vi "NanoStep Goto.vi"(0 "VISA Rsrc":refnum<visa-resource-name>="GPIB1::15::INSTR", 1 "AxeInv":bool, 5 "Position":dbl=0.5, 7 "Input Units":i8(ring) items=["mm", "ps"], 9 "Axis":u16(ring)=1 items=["Axis 0", "Axis 1"], 11 "error in":errorcluster, 12 "CtrlRef":T1 caption="Control Reference") -> (6 "Pos Out":dbl=0.5, 15 "error out":errorcluster)   [LabVIEW 2010]
uses:
  <userlib>/GenProg/WritebyRefBool.vi
  <userlib>/GenProg/ReadbyRefBool.vi
  <userlib>/GenProg/WritebyRefNum.vi
panel:
  in  "Annuler":bool
  out "Init Done":bool
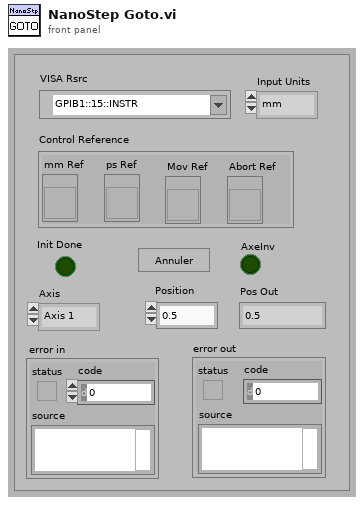
[diagram p1: front panel]
types:
  T1 = cluster{"mm Ref":refnum<vi>, "ps Ref":refnum<vi>, "Mov Ref":refnum<vi>, "Abort Ref":refnum<vi>}
  T2 = enum16{"send command", "Init axis", "read position", "read limit", "end"}
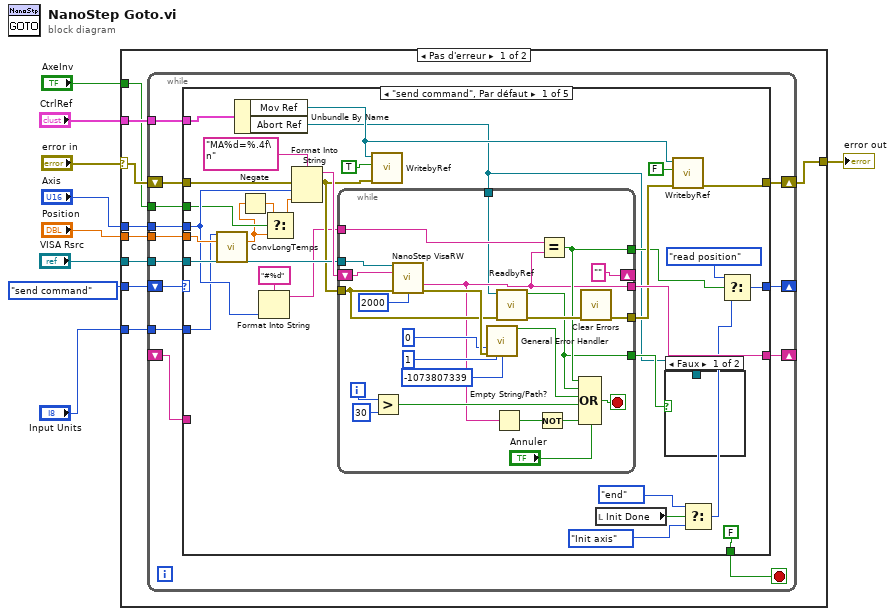
[diagram p0: block diagram]
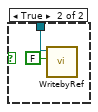
[diagram p2: hidden frame]
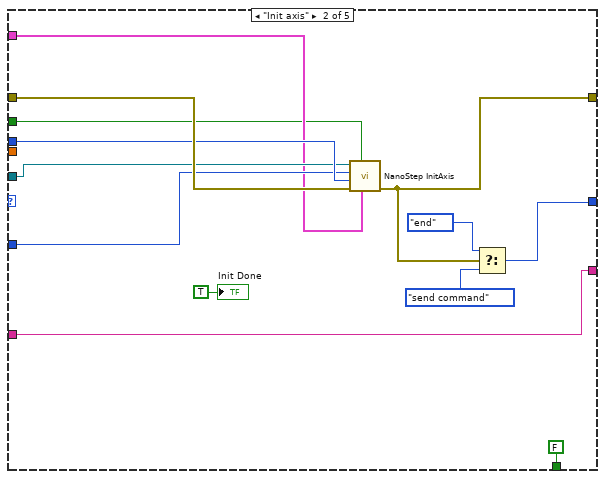
[diagram p3: hidden frame]
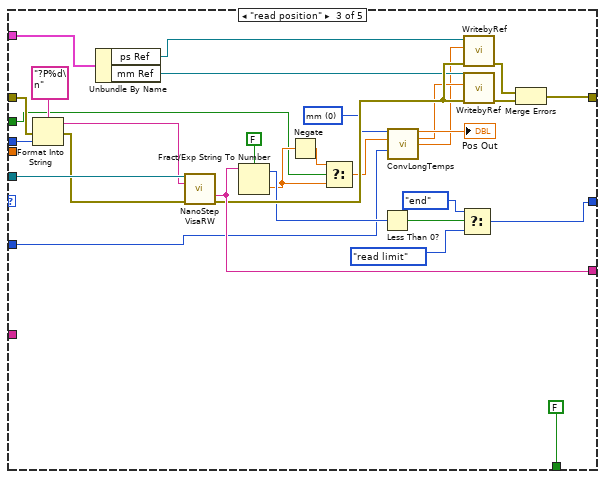
[diagram p4: hidden frame]
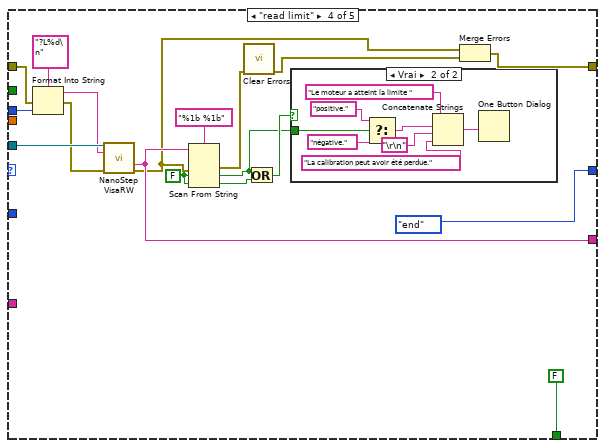
[diagram p5: hidden frame]
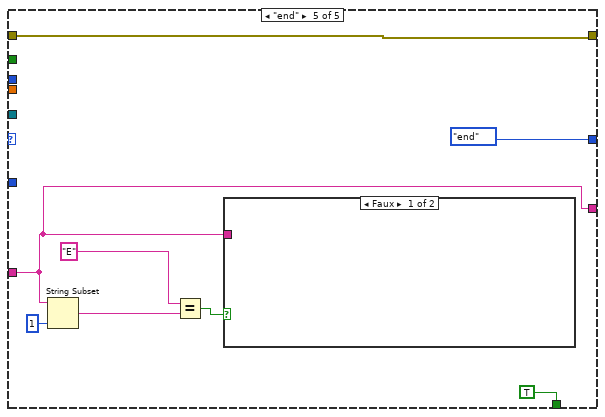
[diagram p7: hidden frame]
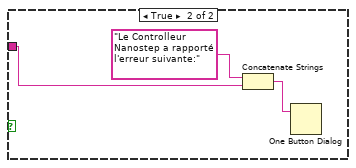
[diagram p8: hidden frame]
diagram:
  n1 = case shown="Pas d'erreur" "error in" {
    selector: "error in" -> [w15 w169]
    tunnel: "Axis" -> [w17 _]
    tunnel: "Position" -> [w18 _]
    tunnel: [w14 w169] -> w6
    tunnel: T2."send command" ("Énum") -> [w16 _]
    tunnel: "VISA Rsrc" -> [w13 _]
    tunnel: "Input Units" -> [w12 _]
    tunnel: "CtrlRef" -> [w11 _]
    tunnel: "AxeInv" -> [w10 _]
    frame No Error {
      n2 = while {
        tunnel: w18 -> [w31]
        tunnel: w17 -> [w30]
        shift-right: [w26] -> w14
        shift-left: w15 -> [w28]
        tunnel: w13 -> [w27]
        shift-right: [w24] -> _
        shift-left: w16 -> [w29]
        shift-right: [w23] -> _
        shift-left: _ -> [w22]
        tunnel: w12 -> [w21]
        tunnel: w11 -> [w20]
        tunnel: w10 -> [w19]
        stop <- w25 stop-if-true
        n3 = case shown="\"send command\", Par défaut" w29 {
          tunnel: w31 -> [w53 _ _ _ _]
          tunnel: w30 -> [w45 w100 w129 w147 _]
          tunnel: w28 -> [w61 w101 w128 w146 w161]
          tunnel: w27 -> [w57 w98 w131 w149 _]
          tunnel: [w51 w97 w120 w137 w161] -> w26
          tunnel: [FALSE FALSE FALSE FALSE TRUE] -> w25
          tunnel: [w58 w96 w114 T2."end" ("Énum") T2."end" ("Énum")] -> w24
          tunnel: [w56 w95 w123 w141 w159] -> w23
          tunnel: w22 -> [_ w95 _ _ w159]
          tunnel: w21 -> [w36 w99 w110 _ _]
          tunnel: w20 -> [w39 w90 w113 _ _]
          tunnel: w19 -> [w35 w89 w103 _ _]
          frame "send command", Default {
            n4 = call <userlib>:"ConvLongTemps.vi"("Input Units"=w36, "Units Input"=w53) -> ("Units mm"=w32:dbl)  [unwired: 10 in, 3 out]
            n5 = Unbundle By Name(w39) -> ("Mov Ref"=w38:refnum<vi>, "Abort Ref"=w37:refnum<vi>)
            n6 = Negate(x=w32) -> (-x=w34:dbl)
            n7 = Format Into String(format string="#%d" ("chaîne de format"), w45) -> (resulting string=w44:string)  [unwired: 2 in, 1 out]
            n8 = Select(t=w34, s=w35, f=w32) -> (s? t:f=w33:dbl)
            n9 = Format Into String(format string="MA%d=%.4f\n", error in=w61, w45, w33) -> (resulting string=w60:string, error out=w49:errorcluster)  [unwired: 1 in]
            n10 = while {
              tunnel: w49 -> [w80]
              tunnel: [w71] -> w52
              tunnel: w57 -> [w87]
              tunnel: [w68] -> w56
              shift-right: [""] -> _
              shift-left: w60 -> [w88]
              tunnel: [w72] -> w47
              tunnel: w44 -> [w67]
              tunnel: [w66] -> w40
              tunnel: w37 -> [w65]
              i -> [w86]
              stop <- w78 stop-if-true
              n11 = Greater?(x=w86, y=30) -> (0:w84:bool)
              n12 = call <userlib>:"NanoStep VisaRW.vi"("VISA Rsrc"=w87, "ChaineCom"=w88, "error in (no error)"=w80, "Timeout(ms)"=u32 2000) -> ("ChaineRep"=w68:string, "error out"=w81:errorcluster)  [unwired: 8 in, 2 out]
              n13 = call <vilib>:"General Error Handler.vi"("type of dialog (OK msg:1)"=u16 0 ("[exception code]"), "error in (no error)"=w81, "[exception action] (none:0)"=1 ("y"), "[exception code]"=-1073807339) -> ("error?"=w79:bool)  [unwired: 7 in, 4 out]
              n14 = Empty String/Path?(string/path=w68) -> (empty?=w70:bool)
              n15 = call-poly <userlib>:"ReadbyRef.vi"("error in"=w80, "Control Ref"=w65) -> ("error out"=w83:errorcluster, "Valeur"=w66:bool)  [unwired: 8 in]
              n16 = Not(x=w70) -> (.not. x?=w69:bool)
              n17 = Equal?(x=w67, y=w68) -> (x = y?=w72:bool)
              n18 = Compound Arithmetic op=OR(w72, w66, w79, w84, "Annuler", w69) -> (w78:bool)
              n19 = call <vilib>:"Clear Errors.vi"("error in (no error)"=w83) -> ("error out"=w71:errorcluster)  [unwired: 6 in]
            }
            n20 = call-poly <userlib>:"WritebyRef.vi"("error in"=w49, "Valeur"=TRUE, "Control Ref"=w38) -> ()  [unwired: 8 in, 1 out]
            n21 = local read "Init Done"() -> (w54:bool)
            n22 = case shown="Faux" w40 {
              tunnel: w37 -> [_ w63]
              frame False {
              }
              frame True {
                n23 = call-poly <userlib>:"WritebyRef.vi"("Valeur"=FALSE, "Control Ref"=w63) -> ()  [unwired: 9 in, 1 out]
              }
            }
            n24 = call-poly <userlib>:"WritebyRef.vi"("error in"=w52, "Valeur"=FALSE, "Control Ref"=w38) -> ("error out"=w51:errorcluster)  [unwired: 8 in]
            n25 = Select(t=T2."end" ("Énum"), s=w54, f=T2."Init axis" ("Énum")) -> (s? t:f=w55:T2)
            n26 = Select(t=T2."read position" ("Énum"), s=w47, f=w55) -> (s? t:f=w58:T2)
          }
          frame "Init axis" {
            n27 = call <userlib>:"NanoStep InitAxis.vi"("CtrlRef"=w90, "AxeInv"=w89, "error in"=w101, "Axis"=w100, "Input Units"=w99, "VISA Rsrc"=w98) -> ("error out"=w97:errorcluster)  [unwired: 4 in, 1 out]
            n28 = Select(t=T2."end" ("Énum"), s=w97, f=T2."send command" ("Énum")) -> (s? t:f=w96:T2)
            "Init Done" <- TRUE ("Init Done")
          }
          frame "read position" {
            w109 = i8 0 items=["mm", "ps"] ("Input Units")
            n29 = Format Into String(format string="?P%d\n", error in=w128, w129) -> (resulting string=w126:string, error out=w127:errorcluster)  [unwired: 1 in]
            n30 = Unbundle By Name(w113) -> ("ps Ref"=w112:refnum<vi>, "mm Ref"=w111:refnum<vi>)
            n31 = call <userlib>:"NanoStep VisaRW.vi"("VISA Rsrc"=w131, "ChaineCom"=w126, "error in (no error)"=w127) -> ("ChaineRep"=w123:string, "error out"=w121:errorcluster)  [unwired: 9 in, 2 out]
            n32 = Fract/Exp String To Number(use system decimal point (T)=FALSE ("utiliser le séparateur décimal du système (V)"), string=w123) -> (offset past number=w118:i32, number=w104:dbl)  [unwired: 2 in]
            n33 = Negate(x=w104) -> (-x=w105:dbl)
            n34 = Select(t=w105, s=w103, f=w104) -> (s? t:f=w102:dbl)
            n35 = Less Than 0?(x=w118) -> (x < 0?=w117:bool)
            n36 = call <userlib>:"ConvLongTemps.vi"("Input Units"=w109, "Units Input"=w102, "Output Units"=w110) -> ("Units Output"=→"Pos Out":dbl, "Units mm"=w107:dbl, "Units ps"=w106:dbl)  [unwired: 9 in, 1 out]
            n37 = Select(t=T2."end" ("Énum"), s=w117, f=T2."read limit" ("Énum")) -> (s? t:f=w114:T2)
            n38 = call-poly <userlib>:"WritebyRef.vi"("error in"=w121, "Valeur"=w106, "Control Ref"=w112) -> ("error out"=w119:errorcluster)  [unwired: 8 in]
            n39 = call-poly <userlib>:"WritebyRef.vi"("error in"=w121, "Valeur"=w107, "Control Ref"=w111) -> ("error out"=w122:errorcluster)  [unwired: 8 in]
            n40 = Merge Errors(w119, w122) -> (w120:errorcluster)
          }
          frame "read limit" {
            w139 = FALSE ("utiliser le séparateur décimal du système (V)")
            n41 = Format Into String(format string="?L%d\n", error in=w146, w147) -> (resulting string=w144:string, error out=w145:errorcluster)  [unwired: 1 in]
            n42 = call <userlib>:"NanoStep VisaRW.vi"("VISA Rsrc"=w149, "ChaineCom"=w144, "error in (no error)"=w145) -> ("ChaineRep"=w141:string, "error out"=w136:errorcluster)  [unwired: 9 in, 2 out]
            n43 = Scan From String(format string="%1b %1b" ("chaîne de format"), input string=w141, error in=w136, default 1=w139, default 2=w139) -> (error out=w138:errorcluster, output 1=w132:bool, output 2=w134:bool)  [unwired: 1 in, 2 out]
            n44 = call <vilib>:"Clear Errors.vi"("error in (no error)"=w138) -> ("error out"=w135:errorcluster)  [unwired: 6 in]
            n45 = Or(x=w132, y=w134) -> (x .or. y?=w133:bool)
            n46 = case shown="Vrai" w133 {
              tunnel: w132 -> [_ w157]
              frame False {
              }
              frame True {
                n47 = Select(t="positive.", s=w157, f="négative.") -> (s? t:f=w152:string)
                n48 = Concatenate Strings("Le moteur a atteint la limite ", w152, "\r\n", "La calibration peut avoir été perdue.") -> (w154:string)
                n49 = One Button Dialog(message=w154) -> ()  [unwired: 1 in, 1 out]
              }
            }
            n50 = Merge Errors(w136, w135) -> (w137:errorcluster)
          }
          frame "end" {
            n51 = String Subset(string=w159, length (rest)=1 ("longueur (reste)")) -> (substring=w163:string)  [unwired: 1 in]
            n52 = Equal?(x="E", y=w163) -> (x = y?=w165:bool)
            n53 = case shown="Faux" w165 {
              tunnel: w159 -> [_ w168]
              frame False {
              }
              frame True {
                n54 = Concatenate Strings("Le Controlleur Nanostep a rapporté l'erreur suivante:", w168) -> (w166:string)
                n55 = One Button Dialog(message=w166) -> ()  [unwired: 1 in, 1 out]
              }
            }
          }
        }
      }
    }
    frame Error {
    }
  }
  "error out" <- w6
